vi "Data length guard.vi"(9 "Max length":i32, 11 "Array":dbl[][](array[numeric])) -> (3 "array w/ subset deleted":dbl[][](array[numeric]))   [LabVIEW 2020]
panel:
  out "size(s)":i32[](array[numeric])
  out "processed size(s)":i32[](array[numeric])
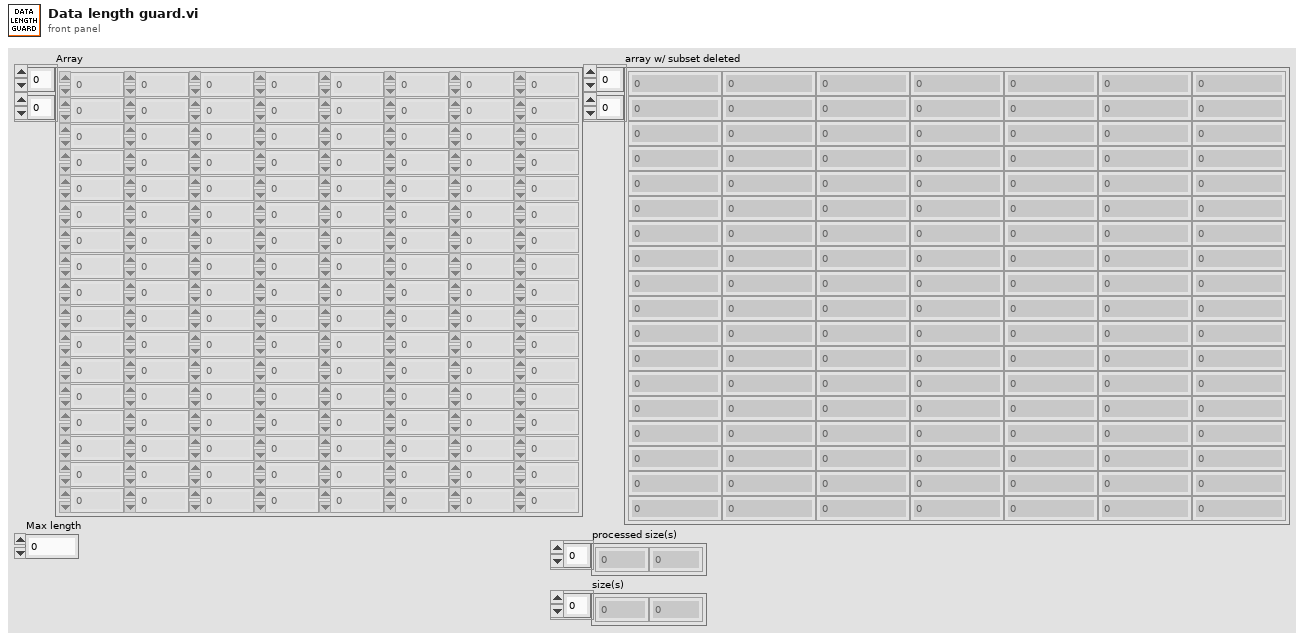
[diagram p1: front panel]
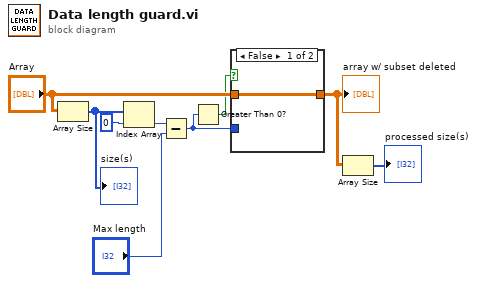
[diagram p0: block diagram]
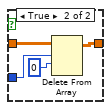
[diagram p2: hidden frame]
diagram:
  n1 = Array Size(array="Array") -> (size(s)=w9:i32[])
  "size(s)" <- w9
  n2 = Index Array(array=w9, index=0) -> (element=w6:i32)
  n3 = Subtract(x=w6, y="Max length") -> (x-y=w3:i32)
  n4 = Greater Than 0?(x=w3) -> (x > 0?=w4:bool)
  n5 = case shown="False" w4 {
    tunnel: "Array" -> [w10 w13]
    tunnel: w3 -> [_ w12]
    tunnel: [w10 w11] -> w2
    frame False {
    }
    frame True {
      n6 = Delete From Array(array=w13, length=w12, index (row)=0) -> (array with subset deleted=w11:dbl[][])  [unwired: 1 in, 1 out]
    }
  }
  "array w/ subset deleted" <- w2
  n7 = Array Size(array=w2) -> (size(s)=→"processed size(s)":i32[])
